vi "Write Channel Setting.vi"(8 "error in (no error)":errorcluster, 10 "Channel Setting":T1={"Address"="None", "SW Alias"="127.0.0.1", "Description"="", "Enabled"=TRUE, "Type"="Type = Class \n"}, 11 "Channel configuration in":refnum<class "Channel configuration.lvclass">) -> (0 "error out":errorcluster, 3 "Channel configuration out":refnum<class "Channel configuration.lvclass">)   [LabVIEW 2025, in "Abstract Engine.lvlib" / "Channel configuration.lvclass"]
uses:
  Channel configuration.lvclass
  Default Channel.ctl
  Channel configuration.lvclass/Channel configuration.ctl
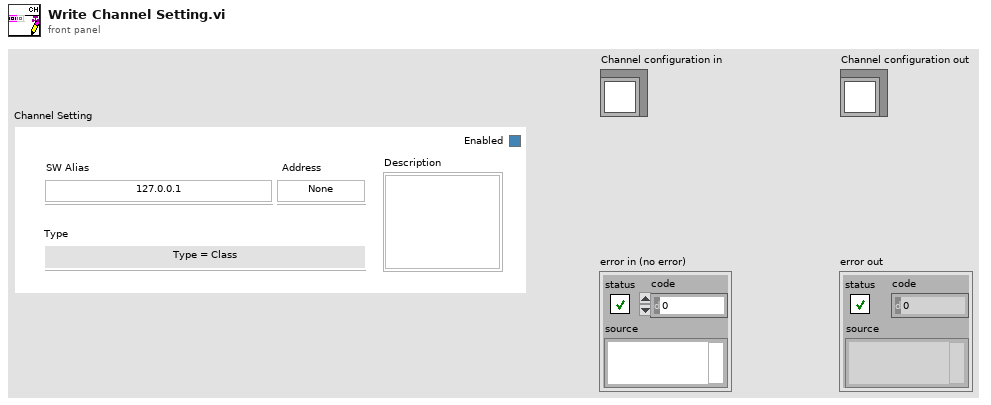
[diagram p1: front panel]
types:
  T1 = typedef "Abstract Engine.lvlib/Channel configuration.lvclass/Default Channel.ctl" = cluster{"Address":string, "SW Alias":string, "Description":string, "Enabled":bool, "Type":string}
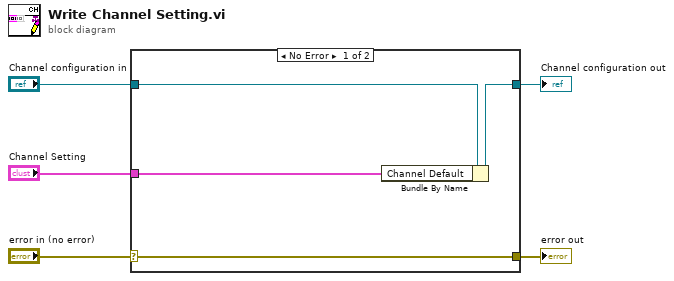
[diagram p0: block diagram]
diagram:
  n1 = case shown="No Error" "error in (no error)" {
    selector: "error in (no error)" -> [w9 w10]
    tunnel: [w9 w10] -> w4
    tunnel: [w7 w11] -> w2
    tunnel: "Channel configuration in" -> [w8 w11]
    tunnel: "Channel Setting" -> [w6 _]
    frame No Error {
      n2 = Bundle By Name(cluster=w8, "Channel Default"=w6) -> (w7:refnum<class "Channel configuration.lvclass">)
    }
    frame Error {
    }
  }
  "error out" <- w4
  "Channel configuration out" <- w2
